vi "SET_HEADING_HIGHPOWER.vi"(10 "argv":string[](array[string]), 11 "args":u8) -> ()   [LabVIEW 2015]
uses:
  Team Code/Robot Global Data.vi
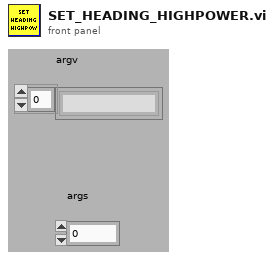
[diagram p1: front panel]
types:
  T1 = cluster{"Yaw":dbl, "Roll":dbl, "Pitch":dbl, "Heading":dbl, "Fused Heading":dbl}
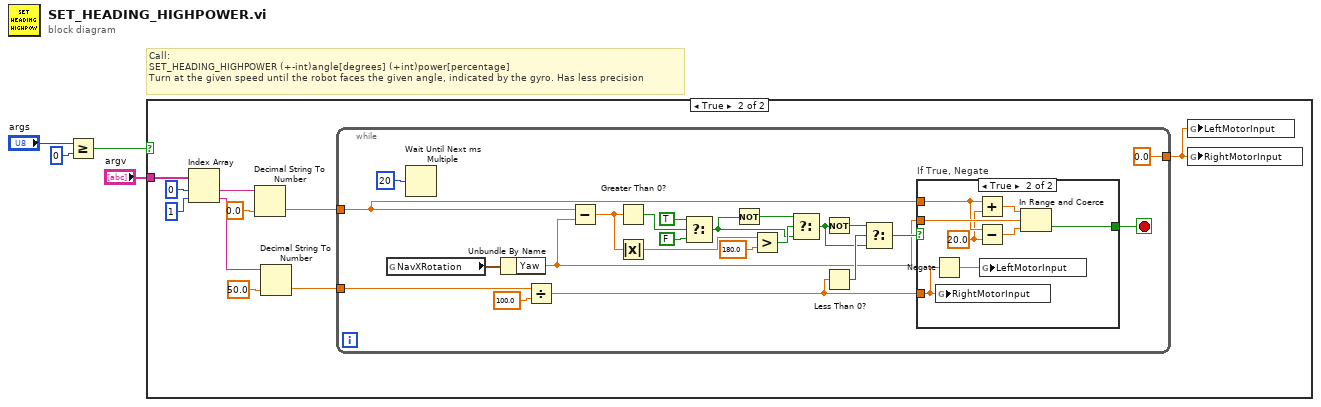
[diagram p0: block diagram]
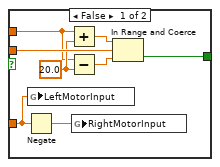
[diagram p3: hidden frame]
diagram:
  # "Call:\nSET_HEADING_HIGHPOWER (+-int)angle[degrees] (+int)power[percentage]\nTurn at the given speed until the robot faces the given angle, indicated by the gyro. Has less precision"
  n1 = Greater Or Equal?(x="args", y=u8 0) -> (x >= y?=w4:bool)
  n2 = case shown="True" w4 {
    tunnel: "argv" -> [_ w7]
    frame False {
    }
    frame True {
      n3 = Index Array(array=w7, index #1=0 ("index"), index #2=1 ("index")) -> (element #1=w8:string, element #2=w6:string)
      n4 = Decimal String To Number(string=w8, default (0L)=0.0 ("default (0 I32)")) -> (number=w9:dbl)  [unwired: 2 out]
      n5 = Decimal String To Number(string=w6, default (0L)=50.0 ("default (0 I32)")) -> (number=w5:dbl)  [unwired: 2 out]
      n6 = while {
        tunnel: w9 -> [w17]
        tunnel: [0.0 ("LeftMotorInput")] -> w14
        tunnel: w5 -> [w32]
        stop <- w35 stop-if-true
        n7 = global read "Robot Global Data.vi" "NavXRotation"() -> (w16:T1)
        n8 = Wait Until Next ms Multiple(millisecond multiple=u32 20) -> ()  [unwired: 1 out]
        n9 = Unbundle By Name(w16) -> ("Yaw"=w15:dbl)
        n10 = Divide(x=w32, y=100.0) -> (x/y=w21:dbl)
        n11 = Subtract(x=w17, y=w15) -> (x-y=w31:dbl)
        n12 = Greater Than 0?(x=w31) -> (x > 0?=w24:bool)
        n13 = Absolute Value(x=w31) -> (abs(x)=w30:dbl)
        n14 = Select(t=TRUE, s=w24, f=FALSE ("s")) -> (s? t:f=w19:bool)
        n15 = Not(x=w19) -> (.not. x?=w20:bool)
        n16 = Greater?(x=w30, y=180.0) -> (0:w23:bool)
        n17 = Select(t=w20, s=w23, f=w19) -> (s? t:f=w18:bool)
        n18 = Not(x=w18) -> (.not. x?=w26:bool)
        n19 = Less Than 0?(x=w21) -> (x < 0?=w22:bool)
        n20 = Select(t=w26, s=w22, f=w18) -> (s? t:f=w25:bool)
        n21 = case "If True, Negate" shown="True" w25 {
          tunnel: w15 -> [w41 w51]
          tunnel: [w42 w52] -> w35
          tunnel: w17 -> [w39 w48]
          tunnel: w21 -> [w38 w45]
          frame False {
            w40 = 20.0
            n22 = Negate(x=w38) -> (-x=w37:dbl)
            n23 = global write "Robot Global Data.vi" "LeftMotorInput"(w38) -> ()
            n24 = Add(x=w39, y=w40) -> (x+y=w44:dbl)
            n25 = Subtract(x=w39, y=w40) -> (x-y=w43:dbl)
            n26 = global write "Robot Global Data.vi" "RightMotorInput"(w37) -> ()
            n27 = In Range and Coerce(upper limit=w44, x=w41, lower limit=w43) -> (In Range?=w42:bool)  [unwired: 1 out]
          }
          frame True {
            w47 = 20.0
            n28 = Negate(x=w45) -> (-x=w46:dbl)
            n29 = global write "Robot Global Data.vi" "RightMotorInput"(w45) -> ()
            n30 = Add(x=w48, y=w47) -> (x+y=w50:dbl)
            n31 = Subtract(x=w48, y=w47) -> (x-y=w49:dbl)
            n32 = global write "Robot Global Data.vi" "LeftMotorInput"(w46) -> ()
            n33 = In Range and Coerce(upper limit=w50, x=w51, lower limit=w49) -> (In Range?=w52:bool)  [unwired: 1 out]
          }
        }
      }
      n34 = global write "Robot Global Data.vi" "LeftMotorInput"(w14) -> ()
      n35 = global write "Robot Global Data.vi" "RightMotorInput"(w14) -> ()
    }
  }
